vi "CheckCameraAttributes-USB3.vi"(2 "error in":errorcluster, 3 "Camera Name":T1) -> (0 "error out":errorcluster, 1 "Session Out":T1)   [LabVIEW 2013]
doc: "The Grab and Attributes Setup VI acquires images continuously and displays the images in an image control using high-level acquisition VIs. The VI also modifes the camera attributes while acquiring images. A grab is appropriate for high-speed applications in which you need to process only one image at a time."
uses:
  <vilib>/userdefined/High Color/IMAQdx.ctl
  <vilib>/vision/driver/IMAQdx.llb/IMAQdx Attribute Type.ctl
  <vilib>/vision/driver/IMAQdx.llb/IMAQdx Attribute Visibility.ctl
  <vilib>/vision/driver/NI_Vision_Acquisition_Software.lvlib
  <resource>/objmgr/imaqdx.rc
panel:
  out "ValueU32":u32
  out "ExposureAuto":string
  out "ExposureCompensation":dbl
  out "Exposure Compensation":string
  out "Debounce Time":i64
  out "Pixel Control On":bool
  out "OverwriteMode":string
  out "SwapPixelBytes":bool
  out "ShiftPixelBits":bool
  out "OutputImageType":string
  out "Timeout":u32
  out "BitsPerPixel":u32(ring) items=["Use Hardware Value"=0, "10-bit"=10, "12-bit"=12, "14-bit"=14, "16-bit"=16]
  out "TestImageSelector":string
  out "PixelSize":string
  out "ReverseX":bool
  out "BinningVertical":i64
  out "VideoMode":string
  out "OffsetY":i64
  out "OffsetX":i64
  out "Height":i64
  out "Width":i64
  out "PixelFormat":string
  out "AcquisitionFrameRateAuto":string
  out "AcquisitionMode":string
  out "ExposureTime":dbl
  out "ExposureMode":string
  out "TriggerActivation":string
  out "TriggerDelayEnabled":bool
  out "TriggerDelay":dbl
  out "TriggerSource":string
  out "TriggerMode":string
  out "TriggerSelector":string
  out "Sharpness":i64
  out "SharpnessEnabled":bool
  out "Gamma":dbl
  out "GammaEnabled":bool
  out "Gain":dbl
  out "GainAuto":string
  out "BlackLevel":dbl
  out "BlackLevelEnabled":bool
  out "Attribute Information Array":T3(array[cluster])
  # "While the values at left are \"Enum\" type, the Property Node only accepts U32 values. \nTo figure out correspondence between number and setting, I had to setup the camera in NIMAX, save the settings (making them defualt) and then use my \"Get Camera Attributes.\""
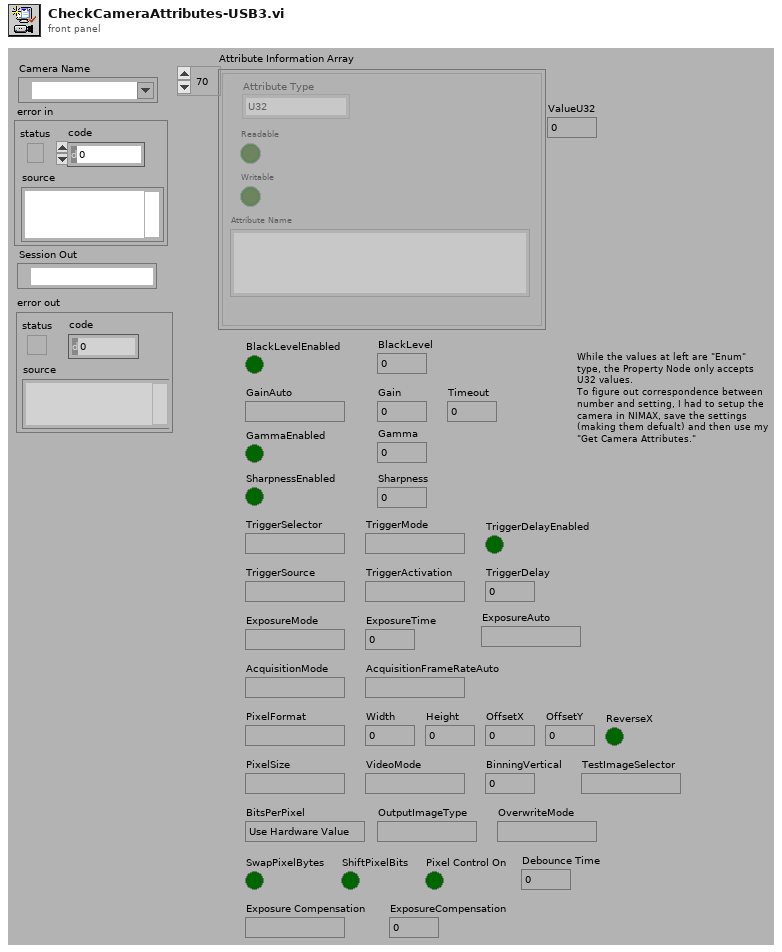
[diagram p1: front panel]
types:
  T1 = typedef "IMAQdx.ctl" = refnum<k21>
  T2 = typedef "NI_Vision_Acquisition_Software.lvlib/IMAQdx Attribute Type.ctl" = enum32{"U32", "I64", "DBL", "String", "Enum", "Bool", "Command"}
  T3 = cluster{"Attribute Type":T2, "Readable":bool, "Writable":bool, "Attribute Name":string}[]
  T4 = typedef "NI_Vision_Acquisition_Software.lvlib/IMAQdx Attribute Visibility.ctl" = enum32{"Simple", "Intermediate", "Advanced"}
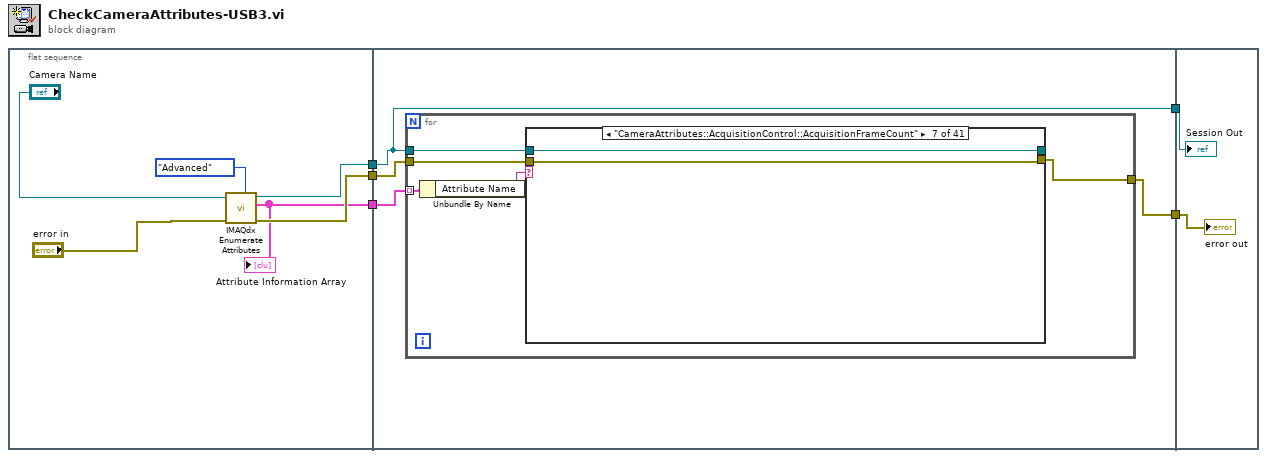
[diagram p0: block diagram]
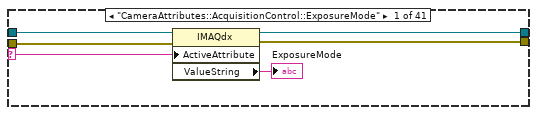
[diagram p2: hidden frame]
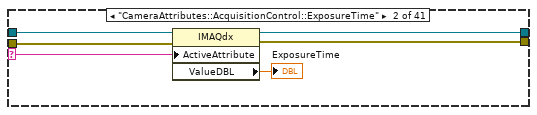
[diagram p3: hidden frame]
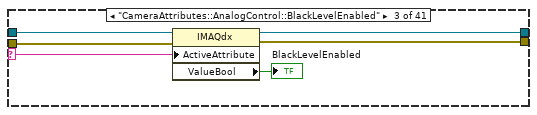
[diagram p4: hidden frame]
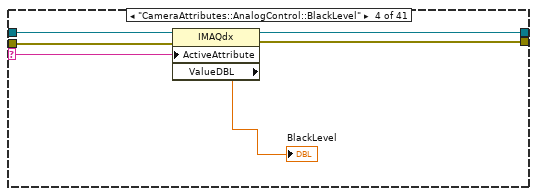
[diagram p5: hidden frame]
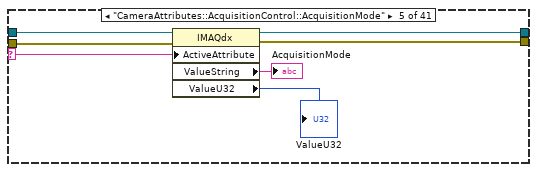
[diagram p6: hidden frame]
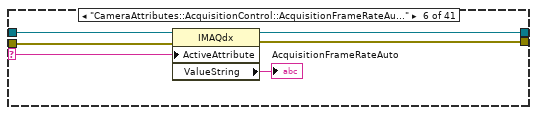
[diagram p7: hidden frame]
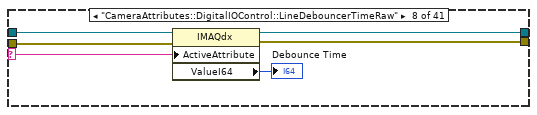
[diagram p8: hidden frame]
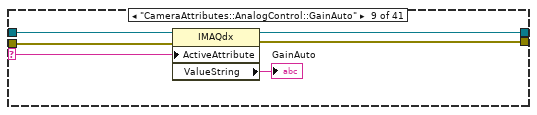
[diagram p9: hidden frame]
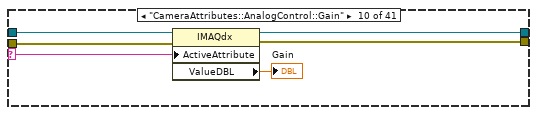
[diagram p10: hidden frame]
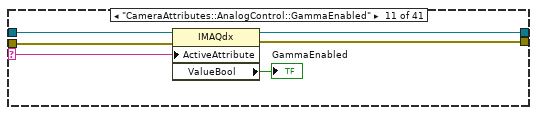
[diagram p11: hidden frame]
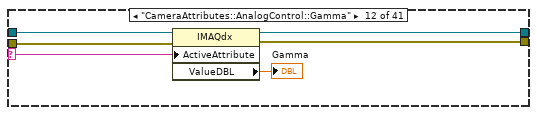
[diagram p12: hidden frame]
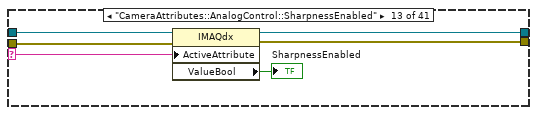
[diagram p13: hidden frame]
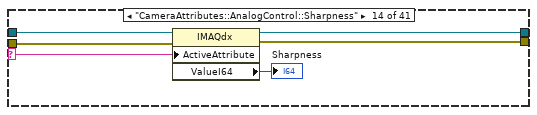
[diagram p14: hidden frame]
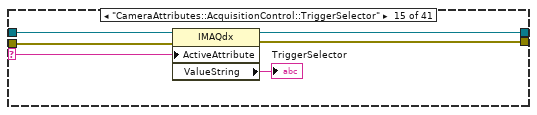
[diagram p15: hidden frame]
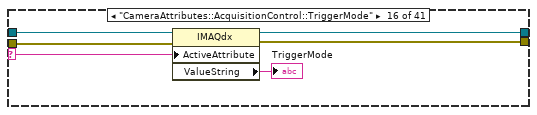
[diagram p16: hidden frame]
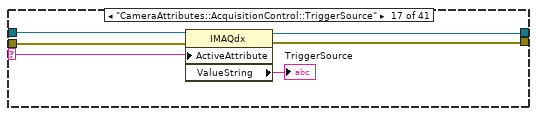
[diagram p17: hidden frame]
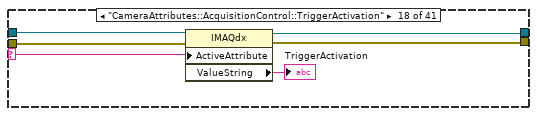
[diagram p18: hidden frame]
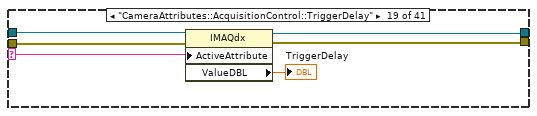
[diagram p19: hidden frame]
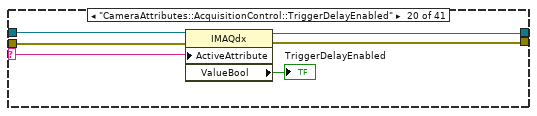
[diagram p20: hidden frame]
diagram:
  n1 = flat-sequence {
    tunnel: [w10] -> w5
    tunnel: [w8] -> w4
    tunnel: [w9] -> w3
    tunnel: w5 -> [w14]
    tunnel: w4 -> [w13]
    tunnel: w3 -> [w15]
    tunnel: [w13] -> w2
    tunnel: [w12] -> w1
    tunnel: w2 -> [w257]
    tunnel: w1 -> [w256]
    frame #0 {
      n2 = call <vilib>:"IMAQdx Enumerate Attributes.vi"("Visibility"=IMAQdx_Attribute_Visibility."Advanced", "error in"="error in", "Session In"="Camera Name") -> ("error out"=w10:errorcluster, "Attribute Information Array"=w9:T3, "Session Out"=w8:T1)  [unwired: 1 in, 5 out]
      "Attribute Information Array" <- w9
    }
    frame #1 {
      n3 = for {
        tunnel: w13 -> [w18]
        tunnel: w14 -> [w17]
        tunnel: w15 -> [w20] mode=indexing
        tunnel: [w16] -> w12
        n4 = Unbundle By Name(w20) -> ("Attribute Name"=w19:string)
        n5 = case shown="\"CameraAttributes::AcquisitionControl::AcquisitionFrameCount\"" w19 {
          selector: w19 -> [w22 w28 w34 w40 w47 w53 _ w61 w67 w73 w79 w85 w91 w97 w103 w109 w117 w123 w129 w135 w139 w145 w151 w157 w163 w169 w176 w181 _ _ w197 w203 _ w214 w220 w226 w232 _ w242 w249 _]
          tunnel: w18 -> [w26 w32 w38 w44 w51 w57 w58 w65 w71 w77 w83 w89 w95 w101 w107 w113 w119 w125 w131 w137 w143 w149 w155 w161 w167 w173 w174 w185 w190 w195 w201 w207 w212 w218 w224 w230 w236 w241 w247 w253 w254]
          tunnel: w17 -> [w25 w31 w37 w43 w50 w56 w59 w64 w70 w76 w82 w88 w94 w100 w106 w112 w118 w124 w130 w136 w142 w148 w154 w160 w166 w172 w175 w184 w189 w194 w200 w206 w211 w217 w223 w229 w235 w240 w246 w252 w255]
          tunnel: [w24 w30 w36 w42 w49 w55 w58 w63 w69 w75 w81 w87 w93 w99 w105 w111 w116 w122 w128 w134 w141 w147 w153 w159 w165 w171 w179 w183 w188 w193 w199 w205 w210 w216 w222 w228 w234 w239 w245 w251 w254] -> _
          tunnel: [w23 w29 w35 w41 w48 w54 w59 w62 w68 w74 w80 w86 w92 w98 w104 w110 w115 w121 w127 w133 w140 w146 w152 w158 w164 w170 w178 w182 w187 w192 w198 w204 w209 w215 w221 w227 w233 w238 w244 w250 w255] -> w16
          frame "CameraAttributes::AcquisitionControl::ExposureMode" {
            n6 = property class="IMAQdx"(reference=w26, error in=w25, "ActiveAttribute"=w22) -> (reference out=w24:T1, error out=w23:errorcluster, "ValueString"=→"ExposureMode":string)
          }
          frame "CameraAttributes::AcquisitionControl::ExposureTime" {
            n7 = property class="IMAQdx"(reference=w32, error in=w31, "ActiveAttribute"=w28) -> (reference out=w30:T1, error out=w29:errorcluster, "ValueDBL"=→"ExposureTime":dbl)
          }
          frame "CameraAttributes::AnalogControl::BlackLevelEnabled" {
            n8 = property class="IMAQdx"(reference=w38, error in=w37, "ActiveAttribute"=w34) -> (reference out=w36:T1, error out=w35:errorcluster, "ValueBool"=→"BlackLevelEnabled":bool)
          }
          frame "CameraAttributes::AnalogControl::BlackLevel" {
            n9 = property class="IMAQdx"(reference=w44, error in=w43, "ActiveAttribute"=w40) -> (reference out=w42:T1, error out=w41:errorcluster, "ValueDBL"=→"BlackLevel":dbl)
          }
          frame "CameraAttributes::AcquisitionControl::AcquisitionMode" {
            n10 = property class="IMAQdx"(reference=w51, error in=w50, "ActiveAttribute"=w47) -> (reference out=w49:T1, error out=w48:errorcluster, "ValueString"=→"AcquisitionMode":string, "ValueU32"=→"ValueU32":u32)
          }
          frame "CameraAttributes::AcquisitionControl::AcquisitionFrameRateAuto" {
            n11 = property class="IMAQdx"(reference=w57, error in=w56, "ActiveAttribute"=w53) -> (reference out=w55:T1, error out=w54:errorcluster, "ValueString"=→"AcquisitionFrameRateAuto":string)
          }
          frame "CameraAttributes::AcquisitionControl::AcquisitionFrameCount" {
          }
          frame "CameraAttributes::DigitalIOControl::LineDebouncerTimeRaw" {
            n12 = property class="IMAQdx"(reference=w65, error in=w64, "ActiveAttribute"=w61) -> (reference out=w63:T1, error out=w62:errorcluster, "ValueI64"=→"Debounce Time":i64)
          }
          frame "CameraAttributes::AnalogControl::GainAuto" {
            n13 = property class="IMAQdx"(reference=w71, error in=w70, "ActiveAttribute"=w67) -> (reference out=w69:T1, error out=w68:errorcluster, "ValueString"=→"GainAuto":string)
          }
          frame "CameraAttributes::AnalogControl::Gain" {
            n14 = property class="IMAQdx"(reference=w77, error in=w76, "ActiveAttribute"=w73) -> (reference out=w75:T1, error out=w74:errorcluster, "ValueDBL"=→"Gain":dbl)
          }
          frame "CameraAttributes::AnalogControl::GammaEnabled" {
            n15 = property class="IMAQdx"(reference=w83, error in=w82, "ActiveAttribute"=w79) -> (reference out=w81:T1, error out=w80:errorcluster, "ValueBool"=→"GammaEnabled":bool)
          }
          frame "CameraAttributes::AnalogControl::Gamma" {
            n16 = property class="IMAQdx"(reference=w89, error in=w88, "ActiveAttribute"=w85) -> (reference out=w87:T1, error out=w86:errorcluster, "ValueDBL"=→"Gamma":dbl)
          }
          frame "CameraAttributes::AnalogControl::SharpnessEnabled" {
            n17 = property class="IMAQdx"(reference=w95, error in=w94, "ActiveAttribute"=w91) -> (reference out=w93:T1, error out=w92:errorcluster, "ValueBool"=→"SharpnessEnabled":bool)
          }
          frame "CameraAttributes::AnalogControl::Sharpness" {
            n18 = property class="IMAQdx"(reference=w101, error in=w100, "ActiveAttribute"=w97) -> (reference out=w99:T1, error out=w98:errorcluster, "ValueI64"=→"Sharpness":i64)
          }
          frame "CameraAttributes::AcquisitionControl::TriggerSelector" {
            n19 = property class="IMAQdx"(reference=w107, error in=w106, "ActiveAttribute"=w103) -> (reference out=w105:T1, error out=w104:errorcluster, "ValueString"=→"TriggerSelector":string)
          }
          frame "CameraAttributes::AcquisitionControl::TriggerMode" {
            n20 = property class="IMAQdx"(reference=w113, error in=w112, "ActiveAttribute"=w109) -> (reference out=w111:T1, error out=w110:errorcluster, "ValueString"=→"TriggerMode":string)
          }
          frame "CameraAttributes::AcquisitionControl::TriggerSource" {
            n21 = property class="IMAQdx"(reference=w119, error in=w118, "ActiveAttribute"=w117) -> (reference out=w116:T1, error out=w115:errorcluster, "ValueString"=→"TriggerSource":string)
          }
          frame "CameraAttributes::AcquisitionControl::TriggerActivation" {
            n22 = property class="IMAQdx"(reference=w125, error in=w124, "ActiveAttribute"=w123) -> (reference out=w122:T1, error out=w121:errorcluster, "ValueString"=→"TriggerActivation":string)
          }
          frame "CameraAttributes::AcquisitionControl::TriggerDelay" {
            n23 = property class="IMAQdx"(reference=w131, error in=w130, "ActiveAttribute"=w129) -> (reference out=w128:T1, error out=w127:errorcluster, "ValueDBL"=→"TriggerDelay":dbl)
          }
          frame "CameraAttributes::AcquisitionControl::TriggerDelayEnabled" {
            n24 = property class="IMAQdx"(reference=w137, error in=w136, "ActiveAttribute"=w135) -> (reference out=w134:T1, error out=w133:errorcluster, "ValueBool"=→"TriggerDelayEnabled":bool)
          }
          frame "CameraAttributes::ImageFormatControl::VideoMode" {
            n25 = property class="IMAQdx"(reference=w143, error in=w142, "ActiveAttribute"=w139) -> (reference out=w141:T1, error out=w140:errorcluster, "ValueString"=→"VideoMode":string)
          }
          frame "CameraAttributes::AcquisitionControl::pgrExposureCompensationAuto" {
            n26 = property class="IMAQdx"(reference=w149, error in=w148, "ActiveAttribute"=w145) -> (reference out=w147:T1, error out=w146:errorcluster, "ValueString"=→"Exposure Compensation":string)
          }
          frame "CameraAttributes::AcquisitionControl::pgrExposureCompensation" {
            n27 = property class="IMAQdx"(reference=w155, error in=w154, "ActiveAttribute"=w151) -> (reference out=w153:T1, error out=w152:errorcluster, "ValueDBL"=→"ExposureCompensation":dbl)
          }
          frame "CameraAttributes::ImageFormatControl::BinningVertical" {
            n28 = property class="IMAQdx"(reference=w161, error in=w160, "ActiveAttribute"=w157) -> (reference out=w159:T1, error out=w158:errorcluster, "ValueI64"=→"BinningVertical":i64)
          }
          frame "CameraAttributes::ImageFormatControl::ReverseX" {
            n29 = property class="IMAQdx"(reference=w167, error in=w166, "ActiveAttribute"=w163) -> (reference out=w165:T1, error out=w164:errorcluster, "ValueBool"=→"ReverseX":bool)
          }
          frame "CameraAttributes::ImageFormatControl::PixelSize" {
            n30 = property class="IMAQdx"(reference=w173, error in=w172, "ActiveAttribute"=w169) -> (reference out=w171:T1, error out=w170:errorcluster, "ValueString"=→"PixelSize":string)
          }
          frame "CameraAttributes::ImageFormatControl::PixelFormat" {
            n31 = property class="IMAQdx"(reference=w174, error in=w175, "ActiveAttribute"=w176) -> (reference out=w179:T1, error out=w178:errorcluster, "ValueString"=→"PixelFormat":string)
          }
          frame "CameraAttributes::ImageFormatControl::TestImageSelector" {
            n32 = property class="IMAQdx"(reference=w185, error in=w184, "ActiveAttribute"=w181) -> (reference out=w183:T1, error out=w182:errorcluster, "ValueString"=→"TestImageSelector":string)
          }
          frame "AcquisitionAttributes::Timeout" {
            n33 = property class="IMAQdx"(reference=w190, error in=w189) -> (reference out=w188:T1, error out=w187:errorcluster, "Timeout"=→"Timeout":u32)
          }
          frame "AcquisitionAttributes::BitsPerPixel" {
            n34 = property class="IMAQdx"(reference=w195, error in=w194) -> (reference out=w193:T1, error out=w192:errorcluster, "BitsPerPixel"=→"BitsPerPixel":u32)
          }
          frame "CameraAttributes::AcquisitionControl::ExposureAuto" {
            n35 = property class="IMAQdx"(reference=w201, error in=w200, "ActiveAttribute"=w197) -> (reference out=w199:T1, error out=w198:errorcluster, "ValueString"=→"ExposureAuto":string)
          }
          frame "AcquisitionAttributes::OutputImageType" {
            n36 = property class="IMAQdx"(reference=w207, error in=w206, "ActiveAttribute"=w203) -> (reference out=w205:T1, error out=w204:errorcluster, "ValueString"=→"OutputImageType":string)
          }
          frame "AcquisitionAttributes::SwapPixelBytes" {
            n37 = property class="IMAQdx"(reference=w212, error in=w211) -> (reference out=w210:T1, error out=w209:errorcluster, "SwapPixelBytes"=→"SwapPixelBytes":bool)
          }
          frame "CameraAttributes::ImageFormatControl::Height" {
            n38 = property class="IMAQdx"(reference=w218, error in=w217, "ActiveAttribute"=w214) -> (reference out=w216:T1, error out=w215:errorcluster, "ValueI64"=→"Height":i64)
          }
          frame "CameraAttributes::ImageFormatControl::Width" {
            n39 = property class="IMAQdx"(reference=w224, error in=w223, "ActiveAttribute"=w220) -> (reference out=w222:T1, error out=w221:errorcluster, "ValueI64"=→"Width":i64)
          }
          frame "CameraAttributes::ImageFormatControl::OffsetX" {
            n40 = property class="IMAQdx"(reference=w230, error in=w229, "ActiveAttribute"=w226) -> (reference out=w228:T1, error out=w227:errorcluster, "ValueI64"=→"OffsetX":i64)
          }
          frame "CameraAttributes::ImageFormatControl::OffsetY" {
            n41 = property class="IMAQdx"(reference=w236, error in=w235, "ActiveAttribute"=w232) -> (reference out=w234:T1, error out=w233:errorcluster, "ValueI64"=→"OffsetY":i64)
          }
          frame "AcquisitionAttributes::ShiftPixelBits" {
            n42 = property class="IMAQdx"(reference=w241, error in=w240) -> (reference out=w239:T1, error out=w238:errorcluster, "ShiftPixelBits"=→"ShiftPixelBits":bool)
          }
          frame "CameraAttributes::ImageFormatControl::PixelDefectControl::pgrDefectPixelCorrectionEnable" {
            n43 = property class="IMAQdx"(reference=w247, error in=w246, "ActiveAttribute"=w242) -> (reference out=w245:T1, error out=w244:errorcluster, "ValueBool"=→"Pixel Control On":bool)
          }
          frame "AcquisitionAttributes::OverwriteMode" {
            n44 = property class="IMAQdx"(reference=w253, error in=w252, "ActiveAttribute"=w249) -> (reference out=w251:T1, error out=w250:errorcluster, "ValueString"=→"OverwriteMode":string)
          }
          frame Default {
          }
        }
      }
    }
    frame #2 {
      "error out" <- w256
      "Session Out" <- w257
    }
  }
